vi "Dec 3.vi"() -> ()   [LabVIEW 2020]
uses:
  <vilib>/Analysis/NI_AALBase.lvlib
  <vilib>/Analysis/3filter.llb/Butterworth Filter (DBL).vi
  <vilib>/Analysis/3filter.llb/Filter Passband Type.ctl
  <vilib>/Utility/file.llb/Write Delimited Spreadsheet (string).vi
  <vilib>/Utility/file.llb/Write Delimited Spreadsheet (DBL).vi
  <vilib>/DAQmx/read.llb/DAQmx Read (Analog 1D DBL NChan 1Samp).vi
  <vilib>/DAQmx/create/channels.llb/DAQmx Create Channel (AI-Voltage-Basic).vi
  <vilib>/DAQmx/configure/timing.llb/DAQmx Timing (Sample Clock).vi
  <vilib>/Utility/error.llb/DialogType.ctl
panel:
  out "Consumer Loop Speed":u32
  out "Producer Loop Speed":u32
  out "Swing":bool
  out "Force Plate":dynamicdata(graph)
  out "Accelerometers":dynamicdata(graph)
  out "Enlapsed Time (sec)":dbl
  in  "Master Stop":bool
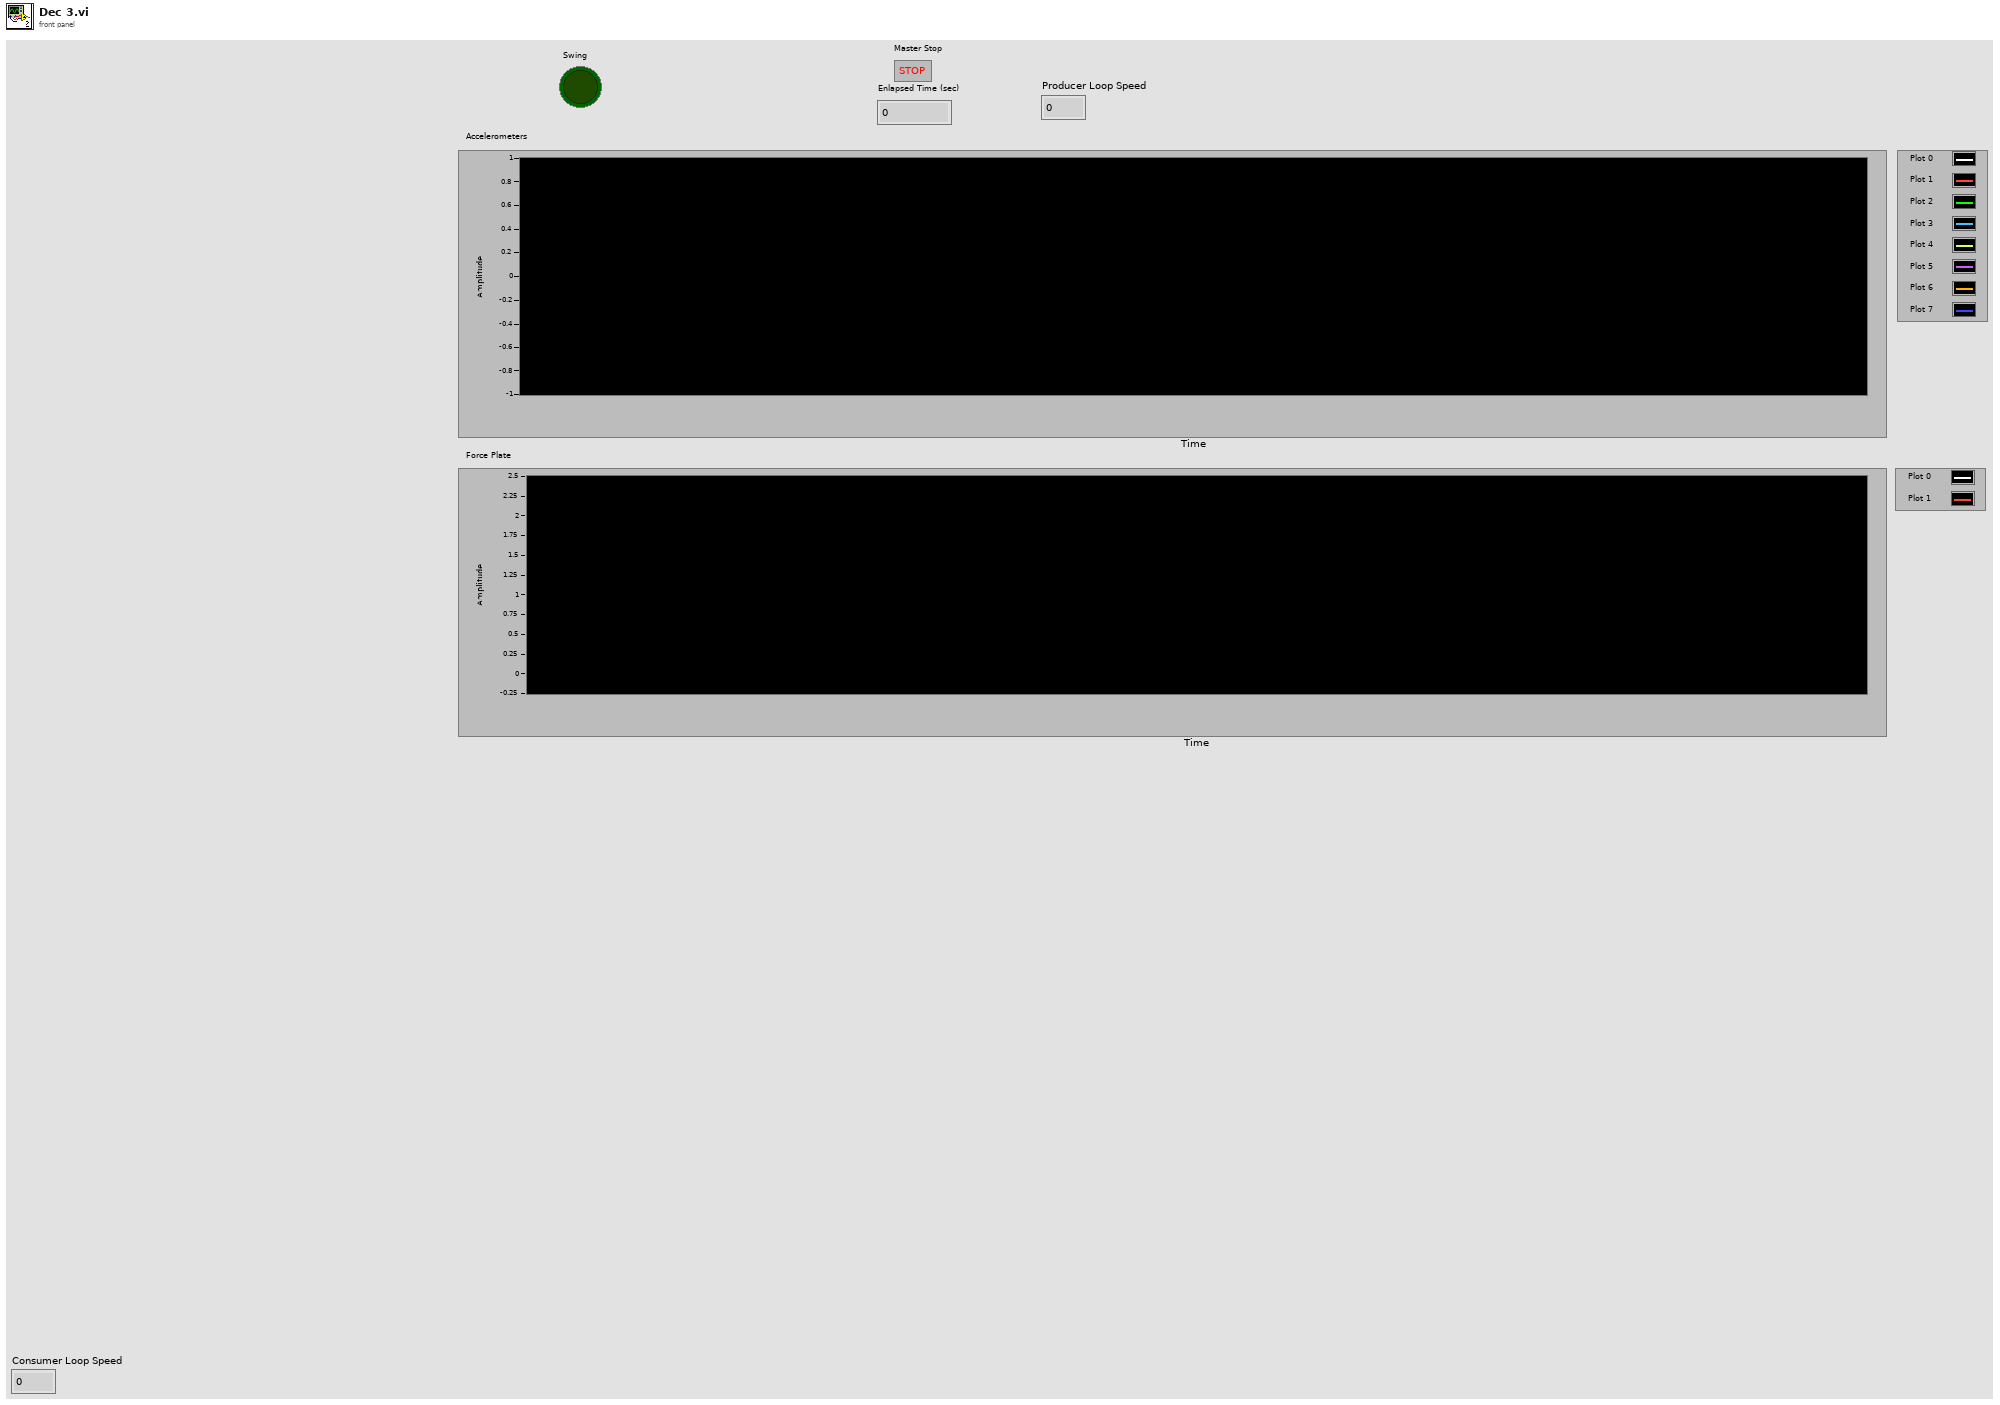
[diagram p1: front panel]
types:
  T1 = typedef "DialogType.ctl" = u16
  T2 = typedef "NI_AALBase.lvlib/Filter Passband Type.ctl" = enum32{"Lowpass", "Highpass", "Bandpass", "Bandstop"}
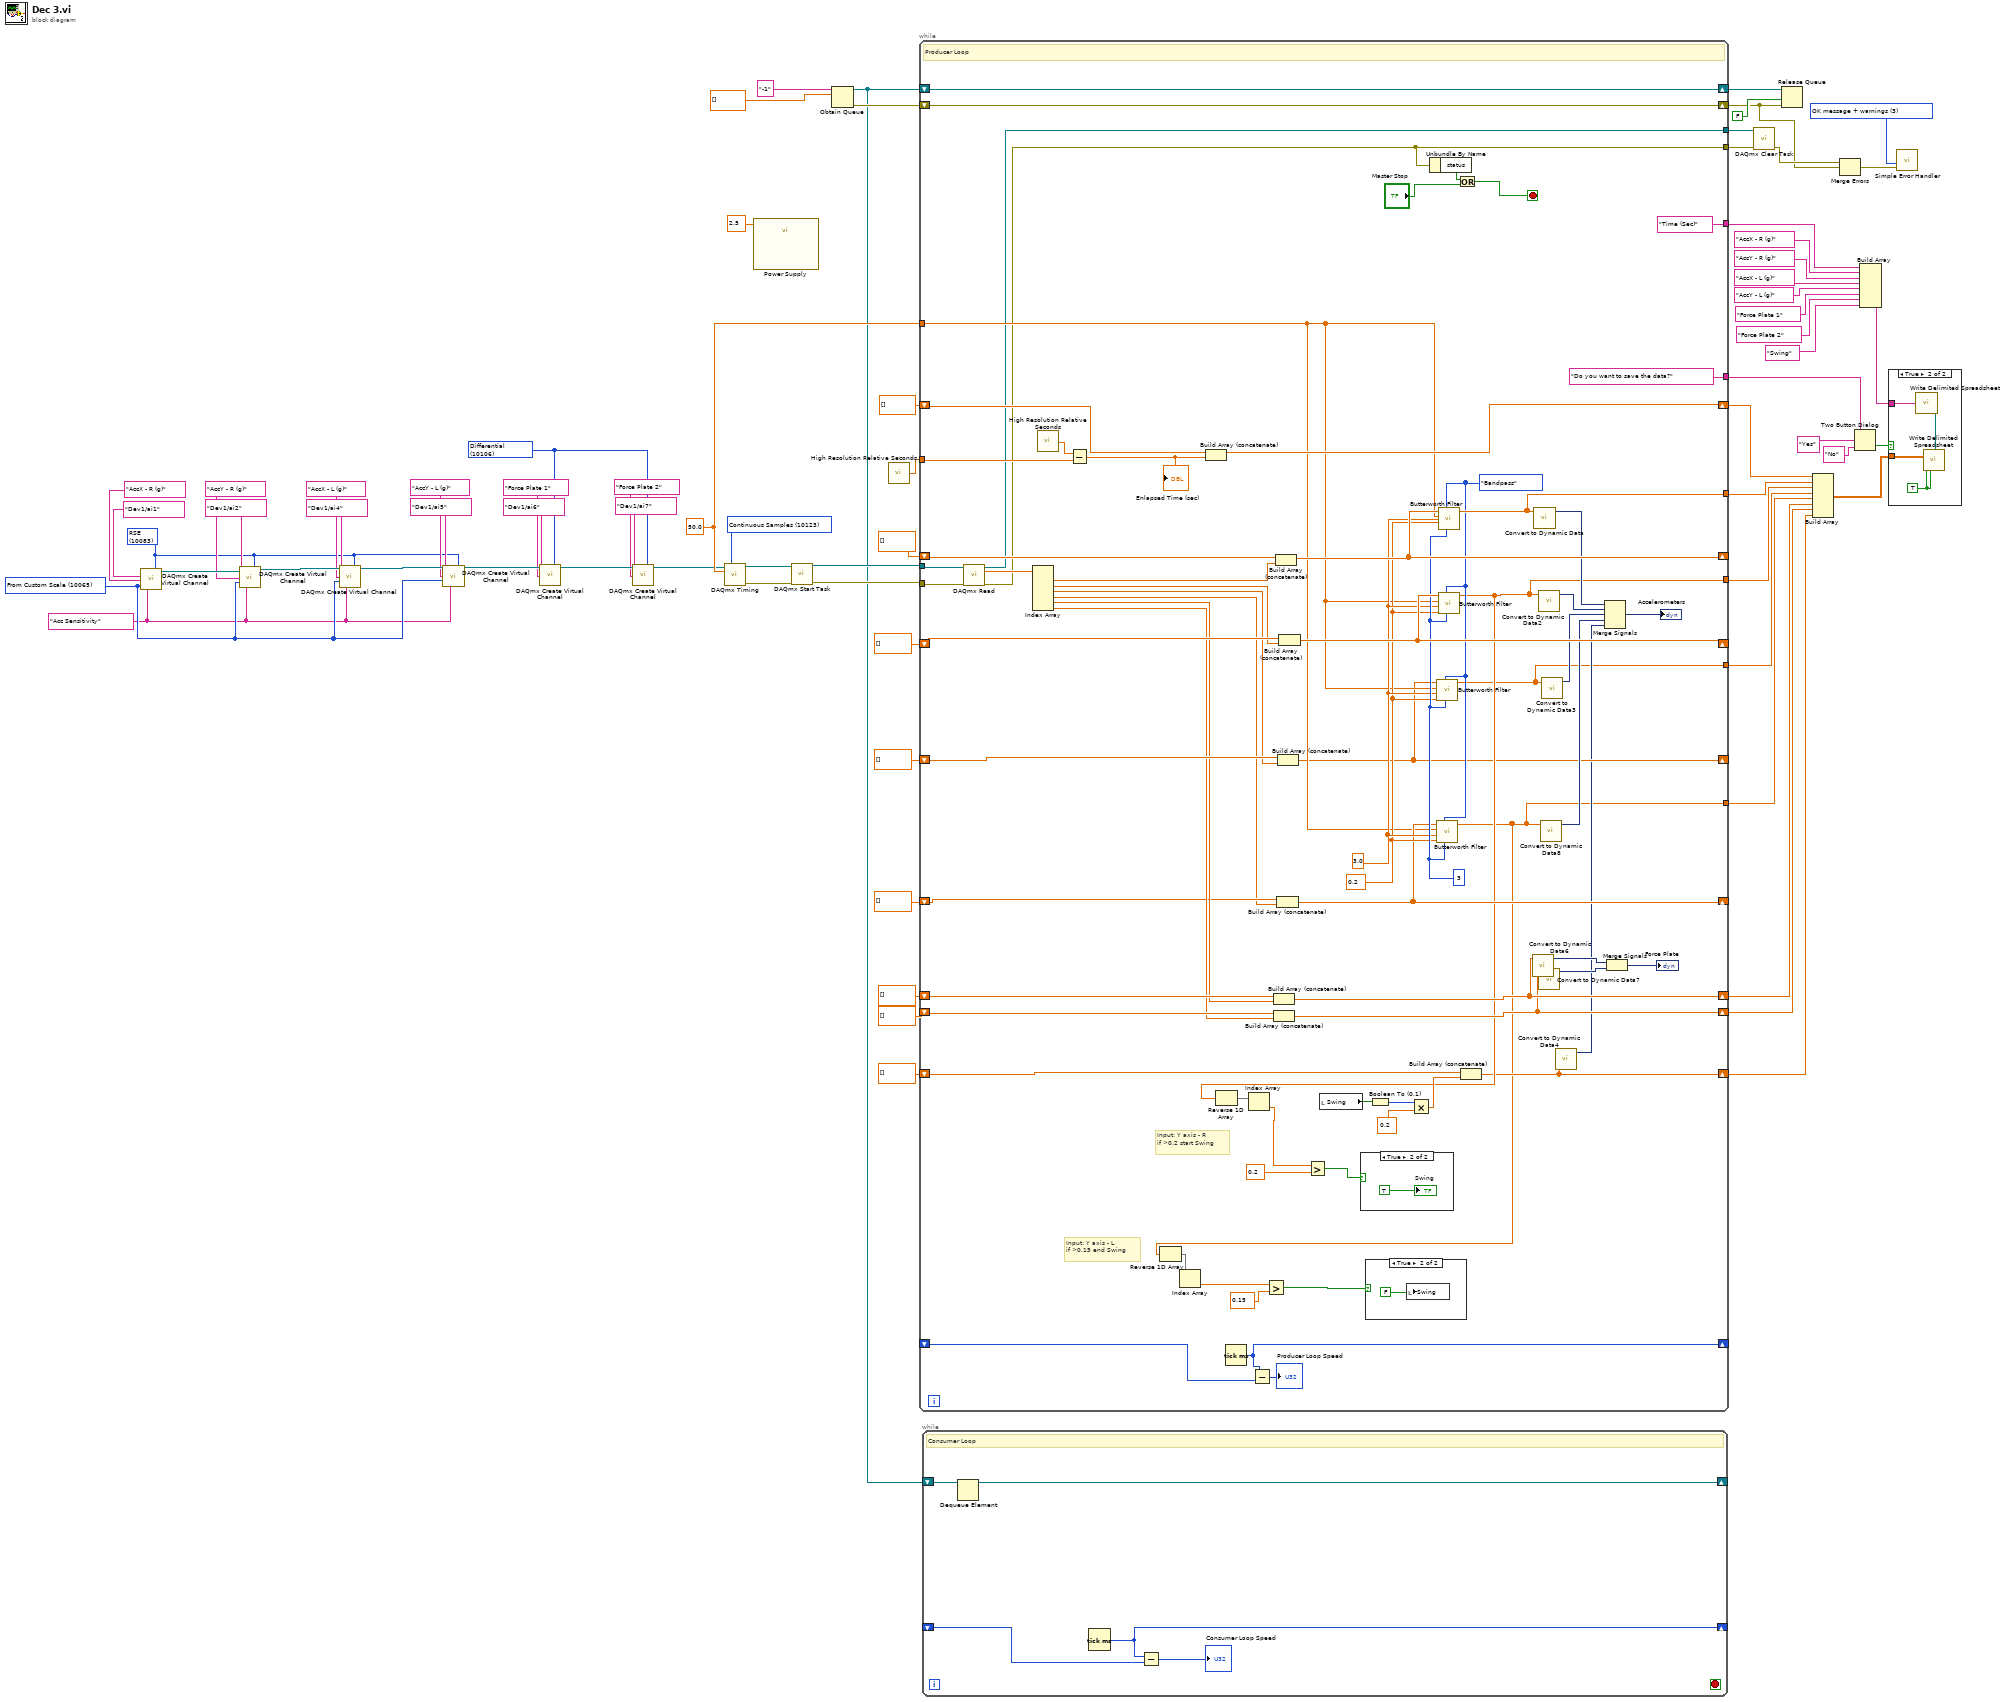
[diagram p0: block diagram]
diagram:
  w5 = T1 3 items=["no dialog", "OK message", "continue or stop message", "OK message + warnings", "continue/stop + warnings"] ("type of dialog (OK msg:1)")
  w16 = 10065 items=["Volts"=10348, "From Custom Scale"=10065] ("units")
  w15 = tag "Acc Sensitivity" ("custom scale name")
  w17 = 10106 items=["Default"=-1, "RSE"=10083, "NRSE"=10078, "Differential"=10106, "Pseudodifferential"=12529] ("input terminal configuration")
  w41 = 10123 items=["Finite Samples"=10178, "Continuous Samples"=10123, "Hardware Timed Single Point"=12522] ("sample mode")
  w36 = 50.0 ("rate")
  w18 = 10083 items=["Default"=-1, "RSE"=10083, "NRSE"=10078, "Differential"=10106, "Pseudodifferential"=12529] ("input terminal configuration")
  n1 = call-poly <vilib>:"DAQmx Create Virtual Channel.vi"("input terminal configuration"=w18, "physical channels"=tag "Dev1/ai1" ("Physical channels"), "name to assign"="AccX - R (g)", "units"=w16, "custom scale name"=w15) -> ("task out"=w35:refnum<k21>)  [unwired: 9 in, 1 out]
  n2 = call-poly <vilib>:"DAQmx Create Virtual Channel.vi"("task in"=w35, "input terminal configuration"=w18, "physical channels"=tag "Dev1/ai2", "name to assign"="AccY - R (g)", "units"=w16, "custom scale name"=w15) -> ("task out"=w34:refnum<k21>)  [unwired: 8 in, 1 out]
  n3 = call-poly <vilib>:"DAQmx Create Virtual Channel.vi"("task in"=w34, "input terminal configuration"=w18, "physical channels"=tag "Dev1/ai4", "name to assign"="AccX - L (g)", "units"=w16, "custom scale name"=w15) -> ("task out"=w33:refnum<k21>)  [unwired: 8 in, 1 out]
  n4 = call-poly <vilib>:"DAQmx Create Virtual Channel.vi"("task in"=w33, "input terminal configuration"=w18, "physical channels"=tag "Dev1/ai5", "name to assign"="AccY - L (g)", "units"=w16, "custom scale name"=w15) -> ("task out"=w32:refnum<k21>)  [unwired: 8 in, 1 out]
  n5 = call-poly <vilib>:"DAQmx Create Virtual Channel.vi"("task in"=w32, "input terminal configuration"=w17, "physical channels"=tag "Dev1/ai6", "name to assign"="Force Plate 1" ("element")) -> ("task out"=w26:refnum<k21>)  [unwired: 10 in, 1 out]
  n6 = call-poly <vilib>:"DAQmx Create Virtual Channel.vi"("task in"=w26, "input terminal configuration"=w17, "physical channels"=tag "Dev1/ai7", "name to assign"="Force Plate 2" ("element")) -> ("task out"=w25:refnum<k21>)  [unwired: 10 in, 1 out]
  n7 = call-poly <vilib>:"DAQmx Timing.vi"("task/channels in"=w25, "sample mode"=w41, "rate"=w36) -> ("task out"=w40:refnum<k21>, "error out"=w39:errorcluster)  [unwired: 11 in]
  n8 = call "Power Supply"("data"=2.5) -> ()  [unwired: 17 in, 2 out]
  n9 = call <vilib>:"DAQmx Start Task.vi"("task/channels in"=w40, "error in"=w39) -> ("task out"=w38:refnum<k21>, "error out"=w37:errorcluster)  [unwired: 12 in]
  n10 = Obtain Queue(name (unnamed)="-1", element data type=dbl[] []) -> (queue out=w1:refnum<queue>, error out=w10:errorcluster)  [unwired: 3 in, 1 out]
  n11 = call <vilib>:"High Resolution Relative Seconds.vi"() -> ("relative seconds"=w72:dbl)
  n12 = while {
    tunnel: w38 -> [w142]
    tunnel: w37 -> [w141]
    tunnel: w72 -> [w139]
    shift-right: [w123] -> w69
    shift-left: dbl[] [] -> [w137]
    shift-right: [w127] -> _
    shift-left: dbl[] [] -> [w136]
    shift-right: [w126] -> _
    shift-left: dbl[] [] -> [w135]
    tunnel: ["Time (Sec)"] -> w44
    tunnel: ["Do you want to save the data?" ("message")] -> w61
    shift-right: [w85] -> w48
    shift-left: dbl[] [] -> [w132]
    shift-right: [w86] -> _
    shift-left: dbl[] [] -> [w124]
    shift-right: [w112] -> w46
    shift-left: dbl[] [] -> [w115]
    shift-right: [w110] -> w47
    shift-left: dbl[] [] -> [w114]
    tunnel: [w108] -> w51
    tunnel: [w89] -> w50
    tunnel: [w81] -> w49
    shift-right: [w101] -> _
    shift-left: dbl[] [] -> [w100]
    tunnel: [w80] -> w45
    tunnel: w36 -> [w98]
    shift-right: [w92] -> _
    shift-left: _ -> [w91]
    shift-right: [w79] -> w9
    shift-left: w1 -> [w79]
    shift-right: [w78] -> w2
    shift-left: w10 -> [w78]
    tunnel: [w77] -> w7
    tunnel: [w73] -> w6
    stop <- w74 stop-if-true
    w105 = 3 ("order")
    w103 = 0.2 ("low cutoff freq: fl")
    w104 = 3.0 ("high cutoff freq: fh")
    w99 = Filter_Passband_Type."Bandpass" ("filter type")
    # "Input: Y axis - L\nif >0.15 end Swing"
    # "Input: Y axis - R\nif >0.2 start Swing"
    # "Producer Loop"
    n13 = call-poly <vilib>:"DAQmx Read.vi"("task/channels in"=w142, "error in"=w141) -> ("task out"=w77:refnum<k21>, "data"=w90:dbl[], "error out"=w73:errorcluster)  [unwired: 11 in]
    n14 = Index Array(array=w90) -> (element #1=w97:dbl, element #2=w96:dbl, element #3=w95:dbl, element #4=w94:dbl, element #5=w106:dbl, element #6=w107:dbl)  [unwired: 6 in]
    n15 = call <vilib>:"High Resolution Relative Seconds.vi"() -> ("relative seconds"=w140:dbl)
    n16 = Subtract(x=w140, y=w139) -> (x-y=w138:dbl)
    "Enlapsed Time (sec)" <- w138
    n17 = Build Array (concatenate)(w137, w138) -> (w123:dbl[])
    n18 = Tick Count (ms)() -> (millisecond timer value=w92:u32)
    n19 = Subtract(x=w92, y=w91) -> (x-y=→"Producer Loop Speed":u32)
    n20 = Build Array (concatenate)(w115, w106) -> (w112:dbl[])
    n21 = Build Array (concatenate)(w114, w107) -> (w110:dbl[])
    n22 = Build Array (concatenate)(w136, w97) -> (w127:dbl[])
    n23 = Build Array (concatenate)(w100, w94) -> (w101:dbl[])
    n24 = Build Array (concatenate)(w124, w95) -> (w86:dbl[])
    n25 = Build Array (concatenate)(w135, w96) -> (w126:dbl[])
    n26 = local read "Swing"() -> (w125:bool)
    n27 = Boolean To (0,1)(Boolean=w125) -> (0, 1=w130:i16)
    n28 = Multiply(x=w130, y=0.2) -> (x*y=w131:dbl)
    n29 = Unbundle By Name(w73) -> ("status"=w76:bool)
    n30 = call-poly <vilib>:"Butterworth Filter.vi"("order"=w105, "filter type"=w99, "low cutoff freq: fl"=w103, "high cutoff freq: fh"=w104, "sampling freq: fs"=w98, "X"=w101) -> ("Filtered X"=w80:dbl[])  [unwired: 2 in, 1 out]
    n31 = Reverse 1D Array(array=w80) -> (reversed array=w117:dbl[])
    n32 = Index Array(array=w117) -> (element=w116:dbl)  [unwired: 1 in]
    n33 = Greater?(x=w116, y=0.15) -> (0:w83:bool)
    n34 = case shown="True" w83 {
      frame False {
      }
      frame True {
        n35 = local write "Swing"(FALSE) -> ()
      }
    }
    n36 = call-poly <vilib>:"Butterworth Filter.vi"("order"=w105, "filter type"=w99, "low cutoff freq: fl"=w103, "high cutoff freq: fh"=w104, "sampling freq: fs"=w98, "X"=w86) -> ("Filtered X"=w81:dbl[])  [unwired: 2 in, 1 out]
    n37 = call-poly <vilib>:"Butterworth Filter.vi"("order"=w105, "filter type"=w99, "low cutoff freq: fl"=w103, "high cutoff freq: fh"=w104, "sampling freq: fs"=w98, "X"=w127) -> ("Filtered X"=w108:dbl[])  [unwired: 2 in, 1 out]
    n38 = call-poly <vilib>:"Butterworth Filter.vi"("order"=w105, "filter type"=w99, "low cutoff freq: fl"=w103, "high cutoff freq: fh"=w104, "sampling freq: fs"=w98, "X"=w126) -> ("Filtered X"=w89:dbl[])  [unwired: 2 in, 1 out]
    n39 = Reverse 1D Array(array=w89) -> (reversed array=w128:dbl[])
    n40 = Index Array(array=w128) -> (element=w88:dbl)  [unwired: 1 in]
    n41 = Greater?(x=w88, y=0.2) -> (0:w82:bool)
    n42 = case shown="True" w82 {
      frame False {
      }
      frame True {
        "Swing" <- TRUE
      }
    }
    n43 = Or(x=w76, y="Master Stop") -> (x .or. y?=w74:bool)
    n44 = Build Array (concatenate)(w132, w131) -> (w85:dbl[])
    n45 = call "Convert to Dynamic Data6"("Array"=w112) -> ("Dynamic Data Type"=w111:dynamicdata)  [unwired: 3 in]
    n46 = call "Convert to Dynamic Data"("Array"=w108) -> ("Dynamic Data Type"=w122:dynamicdata)  [unwired: 3 in]
    n47 = call "Convert to Dynamic Data2"("Array"=w89) -> ("Dynamic Data Type"=w121:dynamicdata)  [unwired: 3 in]
    n48 = call "Convert to Dynamic Data7"("Array"=w110) -> ("Dynamic Data Type"=w109:dynamicdata)  [unwired: 3 in]
    n49 = call "Convert to Dynamic Data8"("Array"=w80) -> ("Dynamic Data Type"=w102:dynamicdata)  [unwired: 3 in]
    n50 = call "Convert to Dynamic Data3"("Array"=w81) -> ("Dynamic Data Type"=w120:dynamicdata)  [unwired: 3 in]
    n51 = call "Convert to Dynamic Data4"("Array"=w85) -> ("Dynamic Data Type"=w84:dynamicdata)  [unwired: 3 in]
    n52 = Merge Signals(w122, w121, w120, w102, w84) -> (→"Accelerometers":dynamicdata)
    n53 = Merge Signals(w111, w109) -> (→"Force Plate":dynamicdata)
  }
  n54 = while {
    shift-right: [w148] -> _
    shift-left: w1 -> [w149]
    shift-right: [w145] -> _
    shift-left: _ -> [w146]
    stop <- _ stop-if-true
    # "Consumer Loop"
    n55 = Dequeue Element(queue=w149) -> (queue out=w148:refnum<queue>)  [unwired: 2 in, 3 out]
    n56 = Tick Count (ms)() -> (millisecond timer value=w145:u32)
    n57 = Subtract(x=w145, y=w146) -> (x-y=→"Consumer Loop Speed":u32)
  }
  n58 = call <vilib>:"DAQmx Clear Task.vi"("task in"=w7, "error in"=w6) -> ("error out"=w3:errorcluster)  [unwired: 13 out]
  n59 = Release Queue(queue=w9, force destroy? (F)=FALSE, error in (no error)=w2) -> ()  [unwired: 3 out]
  n60 = Build Array(w69, w51, w50, w49, w45, w46, w47, w48) -> (w68:dbl[][])
  n61 = Merge Errors(w3, w2) -> (w4:errorcluster)  [unwired: 1 in]
  n62 = Two Button Dialog(message=w61, 1:"No" ("F button name (\"Cancel\")"), 2:"Yes" ("T button name (\"OK\")")) -> (T button?=w64:bool)
  n63 = Build Array(w44, "AccX - R (g)", "AccY - R (g)", "AccX - L (g)", "AccY - L (g)", "Force Plate 1" ("element"), "Force Plate 2" ("element"), "Swing" ("element")) -> (w67:string[])
  n64 = case shown="True" w64 {
    tunnel: w68 -> [_ w153]
    tunnel: w67 -> [_ w152]
    frame False {
    }
    frame True {
      w151 = TRUE ("transpose? (no:F)")
      n65 = call-poly <vilib>:"Write Delimited Spreadsheet.vi"("1D data"=w152) -> ("new file path (Not A Path if cancelled)"=w150:path)  [unwired: 13 in, 1 out]
      n66 = call-poly <vilib>:"Write Delimited Spreadsheet.vi"("file path (dialog if empty)"=w150, "2D data"=w153, "append to file? (new file:F)"=w151, "transpose? (no:F)"=w151) -> ()  [unwired: 10 in, 2 out]
    }
  }
  n67 = call <vilib>:"Simple Error Handler.vi"("type of dialog (OK msg:1)"=w5, "error in (no error)"=w4) -> ()  [unwired: 8 out]
